vi "Tree to Table Array.vi"(7 "Item Indent":u64, 8 "error in (no error)":errorcluster, 10 "Parent UID":string, 11 "Base Tree in":refnum<class "Base Tree.lvclass">) -> (0 "error out":errorcluster, 2 "Tree Items":T1(array[cluster]), 3 "Base Tree out":refnum<class "Base Tree.lvclass">)   [LabVIEW 2017, in "opcua.lvlib" / "Browser Core.lvlib" / "Base Tree.lvclass"]
uses:
  Base Tree.lvclass
  Node Classes/Generic Node/Generic Node.lvclass
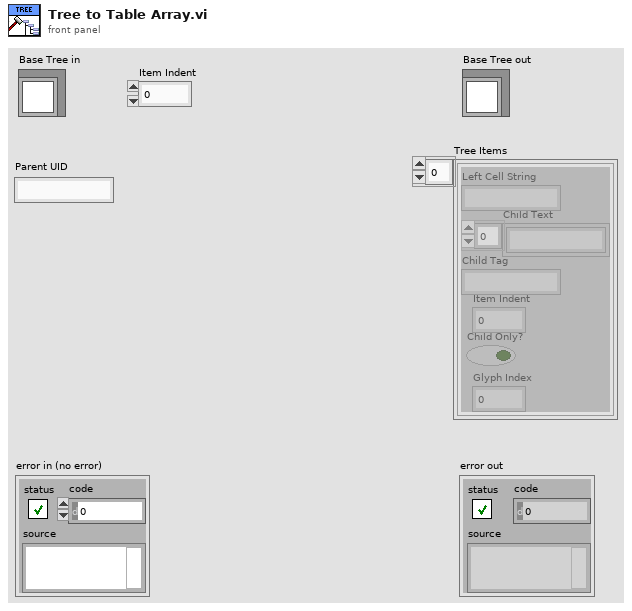
[diagram p1: front panel]
types:
  T1 = cluster{"Left Cell String":string, "Child Text":string[], "Child Tag":string, "Item Indent":i32, "Child Only?":bool, "Glyph Index":i32}[]
  T2 = cluster{"Left Cell String":string, "Child Text":string[], "Child Tag":string, "Item Indent":i32, "Child Only?":bool, "Glyph Index":i32}
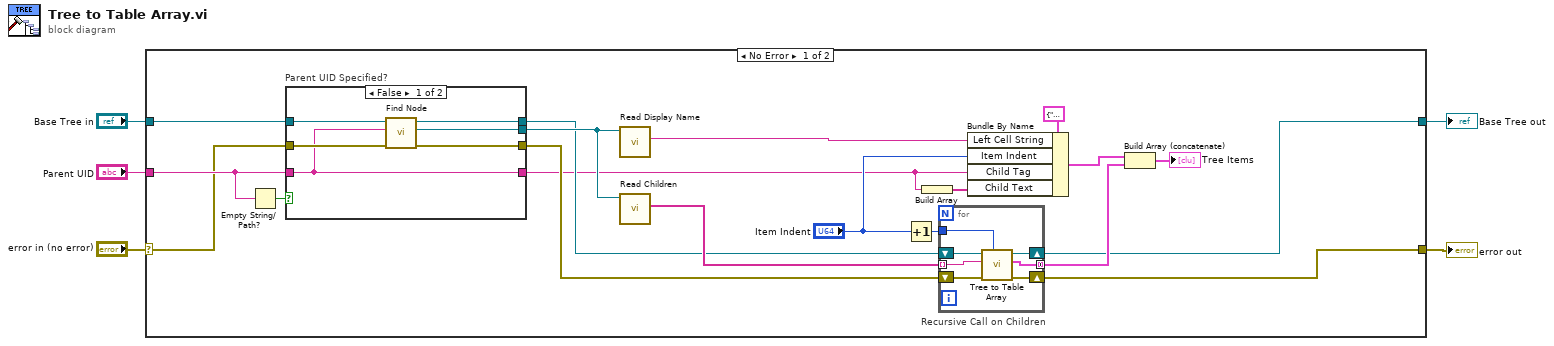
[diagram p0: block diagram]
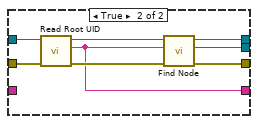
[diagram p2: hidden frame]
diagram:
  n1 = case shown="No Error" "error in (no error)" {
    selector: "error in (no error)" -> [w21 w47]
    tunnel: [w11 w47] -> w4
    tunnel: [w9 w46] -> w2
    tunnel: "Base Tree in" -> [w23 w46]
    tunnel: "Parent UID" -> [w22 _]
    frame No Error {
      n2 = Empty String/Path?(string/path=w22) -> (empty?=w24:bool)
      n3 = case "Parent UID Specified?" shown="False" w24 {
        tunnel: w23 -> [w30 w38]
        tunnel: w22 -> [w25 _]
        tunnel: w21 -> [w29 w35]
        tunnel: [w28 w34] -> w10
        tunnel: [w27 w33] -> w16
        tunnel: [w26 w32] -> w8
        tunnel: [w25 w31] -> w7
        frame False {
          n4 = call-dynamic "Find Node.vi"("error in (no error)"=w29, "UID"=w25, "Base Tree in"=w30) -> ("error out"=w26:errorcluster, "Node"=w27:refnum<class "Generic Node.lvclass">, "Base Tree out"=w28:refnum<class "Base Tree.lvclass">)  [unwired: 5 in, 1 out]
        }
        frame True {
          n5 = call "Read Root UID.vi"("error in (no error)"=w35, "Base Tree in"=w38) -> ("error out"=w36:errorcluster, "Root UID"=w31:string, "Base Tree out"=w37:refnum<class "Base Tree.lvclass">)  [unwired: 7 in]
          n6 = call-dynamic "Find Node.vi"("error in (no error)"=w36, "UID"=w31, "Base Tree in"=w37) -> ("error out"=w32:errorcluster, "Node"=w33:refnum<class "Generic Node.lvclass">, "Base Tree out"=w34:refnum<class "Base Tree.lvclass">)  [unwired: 5 in, 1 out]
        }
      }
      n7 = call "Read Display Name.vi"("Generic Node in"=w16) -> ("Display Name"=w18:string)  [unwired: 8 in, 2 out]
      n8 = call "Read Children.vi"("Generic Node in"=w16) -> ("Children"=w15:string[])  [unwired: 8 in, 2 out]
      n9 = Increment(x="Item Indent") -> (x+1=w14:u64)
      n10 = Build Array(w7) -> (w6:string[])
      n11 = for "Recursive Call on Children" {
        tunnel: w15 -> [w44] mode=indexing
        tunnel: w14 -> [w43]
        tunnel: [w39] -> w13 mode=concatenating
        shift-right: [w41] -> w11
        shift-left: w8 -> [w42]
        shift-right: [w40] -> w9
        shift-left: w10 -> [w45]
        n12 = call-dynamic "Tree to Table Array.vi"("Item Indent"=w43, "error in (no error)"=w42, "Parent UID"=w44, "Base Tree in"=w45) -> ("error out"=w41:errorcluster, "Tree Items"=w39:T1, "Base Tree out"=w40:refnum<class "Base Tree.lvclass">)  [unwired: 5 in]
      }
      n13 = Bundle By Name(cluster=T2 {"Left Cell String"="", "Child Text"=[], "Child Tag"="", "Item Indent"=0, "Child Only?"=FALSE, "Glyph Index"=0} ("Item"), "Left Cell String"=w18, "Item Indent"="Item Indent", "Child Tag"=w7, "Child Text"=w6) -> (w12:T2)
      n14 = Build Array (concatenate)(w12, w13) -> (→"Tree Items":T1)
    }
    frame Error {
    }
  }
  "error out" <- w4
  "Base Tree out" <- w2
